vi "Append Numeric Table to Report.vi"(0 "report in":refnum<class "ooCalc.lvclass">, 1 "column width (1)":dbl=1.0 format="%.2f", 2 "measurement system":u16(ring)=2 caption="measurement system for column width (Default)" items=["US", "Metric", "Default"], 3 "MS Office parameters":T2, 5 "column headers":string[](array[string]), 7 "row headers":string[](array[string]), 9 "numerical data":dbl[][](array[numeric]) format="%.2f", 11 "error in (no error)":errorcluster, 12 "format string (%.3f)":string="%.3f", 13 "separate page?":bool, 14 "show grid lines":bool=TRUE) -> (4 "report out":refnum<class "ooCalc.lvclass">, 8 "range (wd) - start (xl)":T1, 10 "end (xl)":cluster{"row (xl) ":i32, "col (xl) ":i32}, 15 "error out":errorcluster)   [LabVIEW 2009, in "ooCalc.lvclass"]
doc: "Appends a 2D array to a report as a table with the given column width. You can use this polymorphic VI to append an array of strings or numbers. The data type you wire to the <B>text data</B> input determines the polymorphic instance to use."
uses:
  ooCalc.lvclass
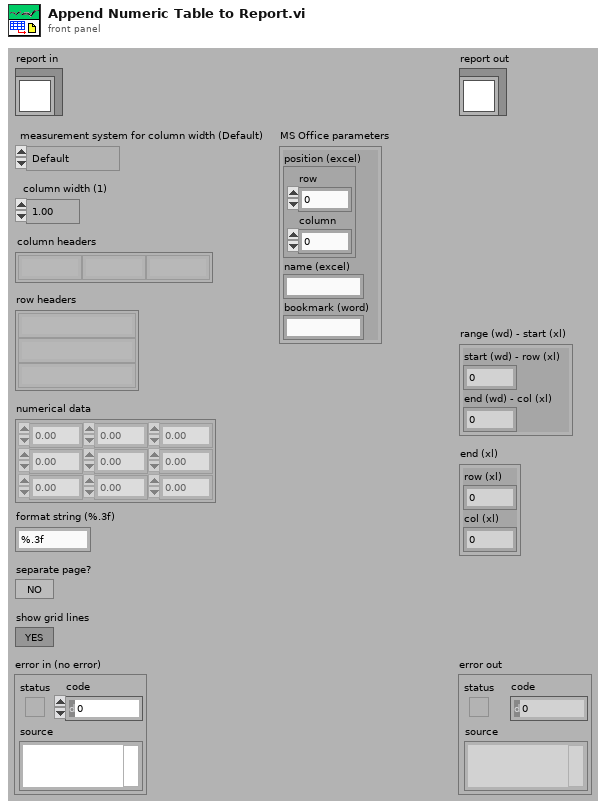
[diagram p1: front panel]
types:
  T1 = cluster{"start (wd) - row (xl) ":i32, "end (wd) - col (xl) ":i32}
  T2 = cluster{"position (excel)":cluster{"row":i32, "column":i32}, "name (excel)":string, "bookmark (word)":string}
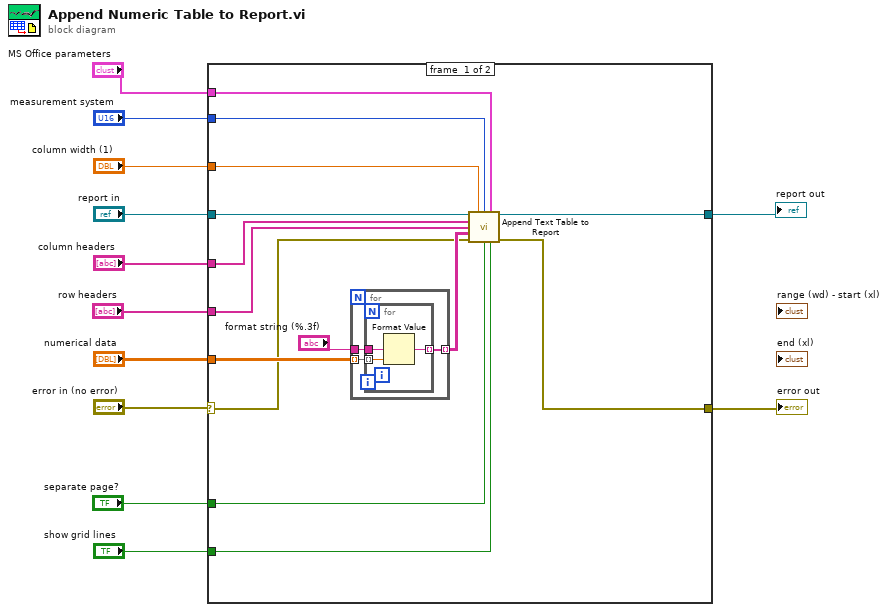
[diagram p0: block diagram]
diagram:
  n1 = case shown="No Error" "error in (no error)" {
    selector: "error in (no error)" -> [w13 w33]
    tunnel: "report in" -> [w26 w34]
    tunnel: [w25 w34] -> w10
    tunnel: [w14 w33] -> w9
    tunnel: "column headers" -> [w24 _]
    tunnel: "row headers" -> [w23 _]
    tunnel: "column width (1)" -> [w20 _]
    tunnel: "measurement system" -> [w19 _]
    tunnel: "MS Office parameters" -> [w18 _]
    tunnel: "separate page?" -> [w17 _]
    tunnel: "show grid lines" -> [w16 _]
    tunnel: "numerical data" -> [w15 _]
    frame #0 {
      n2 = for {
        tunnel: w15 -> [w29] mode=indexing
        tunnel: "format string (%.3f)" -> [w28]
        tunnel: [w27] -> w21 mode=indexing
        n3 = for {
          tunnel: w29 -> [w32] mode=indexing
          tunnel: w28 -> [w31]
          tunnel: [w30] -> w27 mode=indexing
          n4 = Format Value(format string=w31, value (0)=w32) -> (output string=w30:string)  [unwired: 1 in]
        }
      }
      n5 = call-dynamic "Append Text Table to Report.vi"("report in"=w26, "column width (1)"=w20, "measurement system"=w19, "MS Office parameters"=w18, "column headers"=w24, "row headers"=w23, "text data"=w21, "error in (no error)"=w13, "separate page?"=w17, "show grid lines"=w16) -> ("report out"=w25:refnum<class "ooCalc.lvclass">, "error out"=w14:errorcluster)  [unwired: 2 in, 2 out]
    }
    frame #1 {
    }
  }
  "error out" <- w9
  "report out" <- w10
